vi "ZM_valve_state.vi"(0 "Z_Source":T1(ring), 1 "Z_State":T2(ring), 2 "open":bool, 3 "close":bool, 7 "T_start_delay":u32=300, 9 "T_stop_delay":u32=300, 11 "T_restart_delay":u32=3000) -> (14 "Start":bool, 15 "Stop":bool, 16 "End":bool, 17 "ZM_State":u32, 18 "t":u32)   [LabVIEW 2019, in "Valves.lvlib"]
uses:
  Valves.lvlib
  Trigers/RS.vi
  Timer Delay/Timer.vi
  Userlib.lvlib
panel:
  in  "t2_tmp":u32[][](array[numeric])=[[0, 0], [0, 0], [0, 0], [0, 0], [0, 0], [0, 0], [0, 0], [0, 0], [0, 0], [0, 0], [0, 0], [0, 0], [0, 0]]
  in  "C2_tmp":cluster{"C":bool, "NC":u32}[][](array[cluster])
  in  "t_tmp":u32[][](array[numeric])=[[0, 0], [0, 0], [0, 0], [0, 0], [0, 0], [0, 0], [0, 0], [0, 0], [0, 0], [0, 0], [0, 0], [0, 0], [0, 0]]
  in  "C_tmp":cluster{"C":bool, "NC":u32}[][](array[cluster])
  # "Temporally arrays"
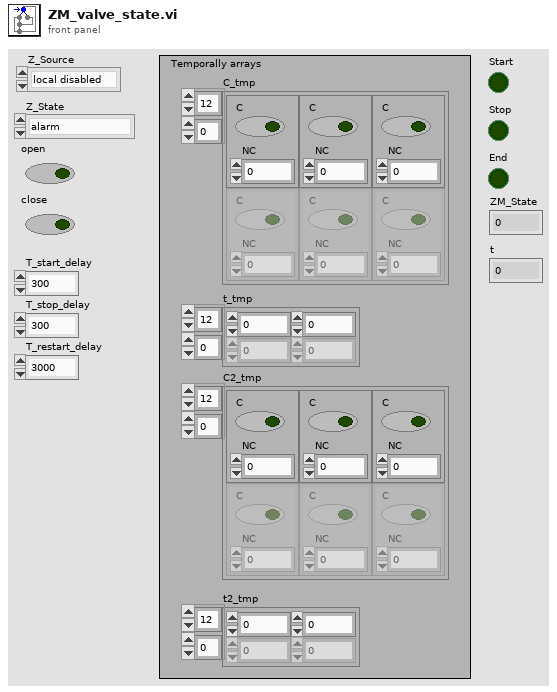
[diagram p1: front panel]
types:
  T1 = enum8{"local disabled", "local hand", "hand", "auto", "dist"}
  T2 = enum8{"alarm", "disabled", "not ready", "stop ready", "reserv", "switched off", "switched on", "check", "on min", "decrease speed", "on", "increase speed", "on max"}
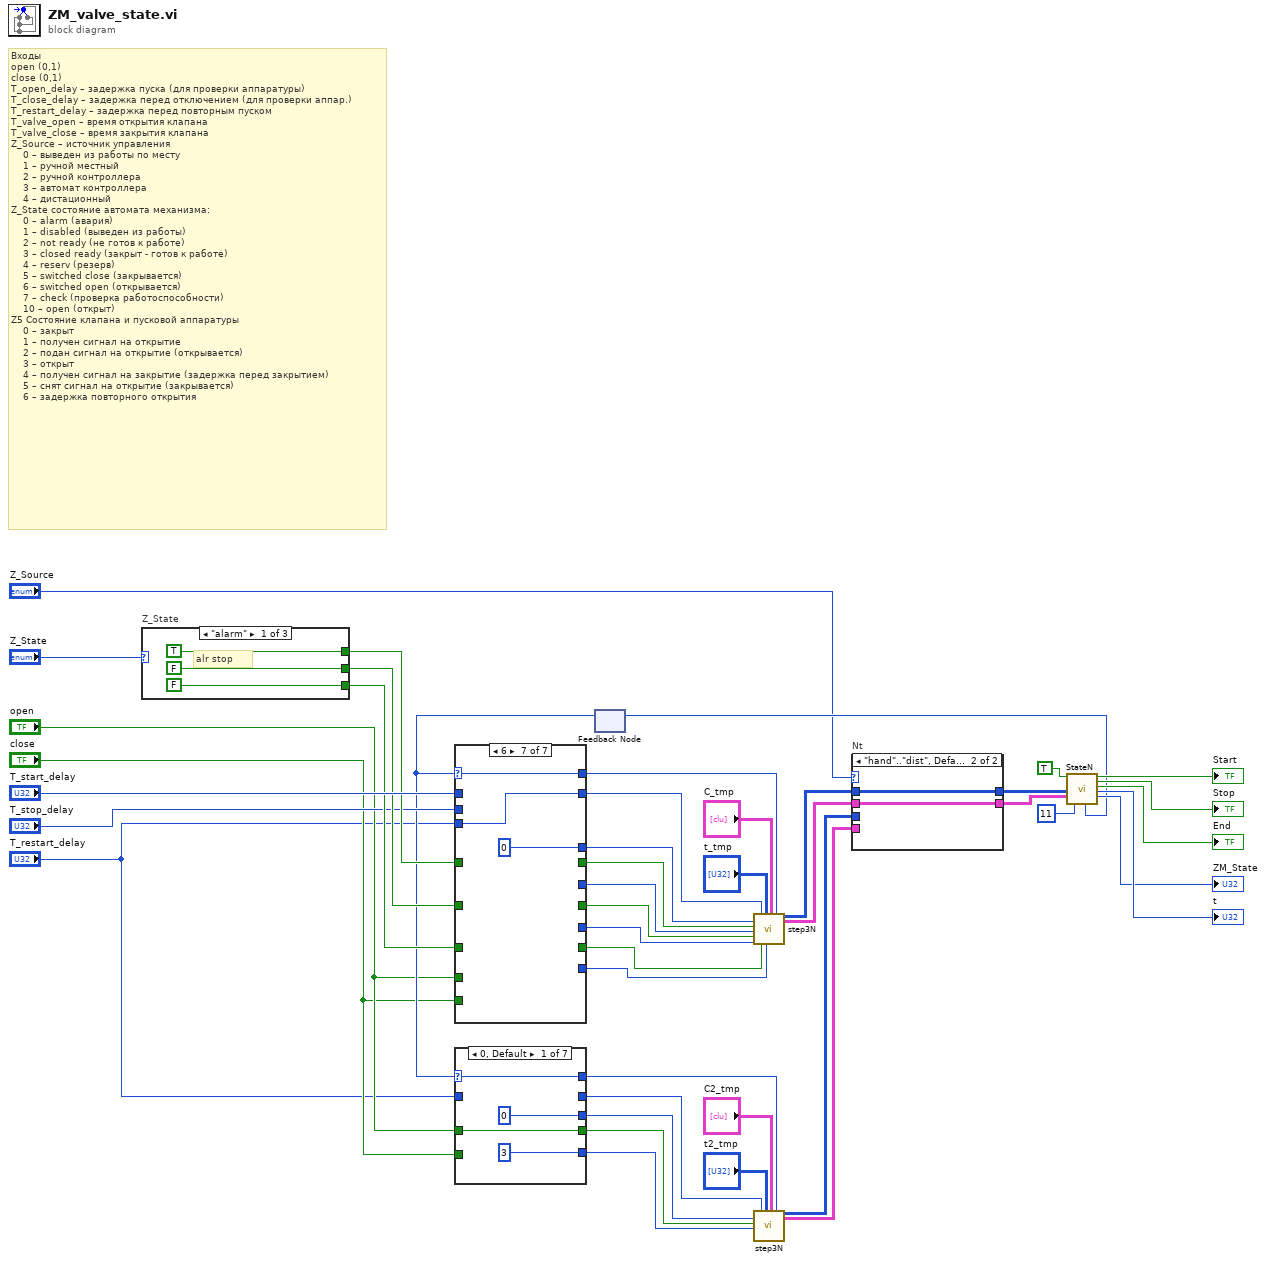
[diagram p0: block diagram]
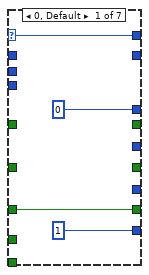
[diagram p2: hidden frame]
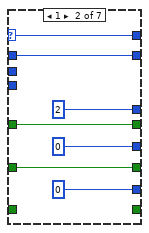
[diagram p3: hidden frame]
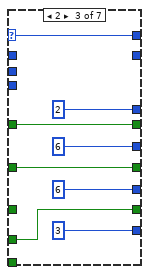
[diagram p4: hidden frame]
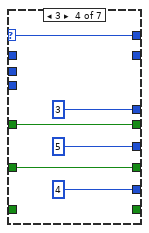
[diagram p5: hidden frame]
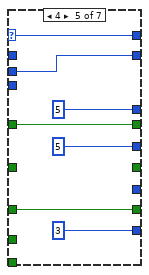
[diagram p6: hidden frame]
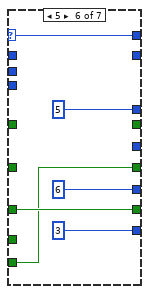
[diagram p7: hidden frame]
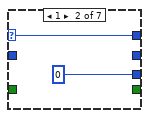
[diagram p8: hidden frame]
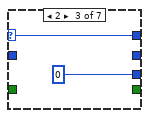
[diagram p9: hidden frame]
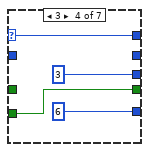
[diagram p10: hidden frame]
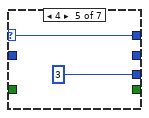
[diagram p11: hidden frame]
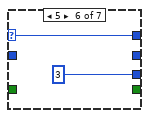
[diagram p12: hidden frame]
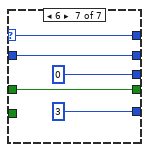
[diagram p13: hidden frame]
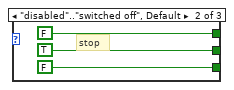
[diagram p15: hidden frame]
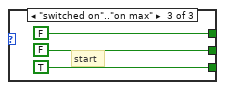
[diagram p16: hidden frame]
diagram:
  # "Входы\nopen (0,1)\nclose (0,1)\nT_open_delay – задержка пуска (для проверки аппаратуры)\nT_close_delay – задержка перед отключением (для проверки аппар.)\nT_restart_delay – задержка перед повторным пуском\nT_valve_open – время открытия клапана\nT_valve_close – время закрытия клапана\nZ_Source – источник управления\n    0 – выведен из работы по месту\n    1 – ручной местный\n    2 – ручной контроллера\n    3 – автомат контроллера\n    4 – дистационный\nZ_State состояние автомата механизма:\n    0 – alarm (авария)\n    1 – disabled (выведен из работы)\n    2 – not ready (не готов к работе)\n    3 – closed ready (закрыт - готов к работе)\n    4 – reserv (резерв)\n    5 – switched close (закрывается)\n    6 – switched open (открывается)\n    7 – check (проверка работоспособности)\n    10 – open (открыт)\nZ5 Состояние клапана и пусковой аппаратуры\n    0 – закрыт\n    1 – получен сигнал на открытие\n    2 – подан сигнал на открытие (открывается)\n    3 – открыт\n    4 – получен сигнал на закрытие (задержка перед закрытием)\n    5 – снят сигнал на открытие (закрывается)\n    6 – задержка повторного открытия"
  n1 = case "Z_State" shown="\"alarm\"" "Z_State" {
    tunnel: [FALSE TRUE FALSE] -> w25
    tunnel: [FALSE FALSE TRUE] -> w27
    tunnel: [TRUE FALSE FALSE] -> w24
    frame "alarm" {
      # "alr stop"
    }
    frame "disabled".."switched off", Default {
      # "stop"
    }
    frame "switched on".."on max" {
      # "start"
    }
  }
  n2 = feedback #1() -> (w11:u32)  [unwired: 1 in]
  n3 = case shown="6" w11 {
    selector: w11 -> [w56 w63 w71 w77 w84 w90 w93]
    tunnel: "T_start_delay" -> [_ w57 _ _ _ _ _]
    tunnel: [w56 w63 w71 w77 w84 w90 w93] -> w20
    tunnel: [u32 0 ("End step") u32 2 ("End step") u32 2 ("End step") u32 3 ("End step") u32 5 ("End step") u32 5 ("End step") u32 0 ("End step")] -> w32
    tunnel: [_ w57 _ _ w78 _ w91] -> w31
    tunnel: [_ w59 w66 w73 w81 _ _] -> w30
    tunnel: [_ u32 0 ("End step") u32 6 ("End step") u32 5 ("End step") u32 5 ("End step") _ _] -> w29
    tunnel: [w54 _ w64 _ w79 w86 _] -> w28
    tunnel: w27 -> [w54 _ _ _ w79 w86 _]
    tunnel: [u32 1 ("End step") _ u32 3 ("End step") _ u32 3 ("End step") u32 3 ("End step") _] -> w26
    tunnel: w25 -> [_ w61 w68 w75 _ _ _]
    tunnel: [_ w61 w68 w75 _ w85 _] -> w23
    tunnel: [_ u32 0 ("End step") u32 6 ("End step") u32 4 ("End step") _ u32 6 ("End step") _] -> w22
    tunnel: w24 -> [_ w59 w66 w73 w81 _ _]
    tunnel: "open" -> [_ _ w64 _ _ _ _]
    tunnel: "T_stop_delay" -> [_ _ _ _ w78 _ _]
    tunnel: "close" -> [_ _ _ _ _ w85 _]
    tunnel: "T_restart_delay" -> [_ _ _ _ _ _ w91]
    frame 0, Default {
    }
    frame 1 {
    }
    frame 2 {
    }
    frame 3 {
    }
    frame 4 {
    }
    frame 5 {
    }
    frame 6 {
    }
  }
  n4 = case shown="0, Default" w11 {
    selector: w11 -> [w97 w99 w101 w105 w107 w109 w114]
    tunnel: [w97 w99 w101 w105 w107 w109 w114] -> w16
    tunnel: [u32 0 ("End step") u32 0 ("End step") u32 0 ("End step") u32 3 ("End step") u32 3 ("End step") u32 3 ("End step") u32 0 ("End step")] -> w12
    tunnel: [_ _ _ _ _ _ w112] -> w13
    tunnel: [w95 _ _ w102 _ _ w111] -> w14
    tunnel: [u32 3 ("End step") _ _ u32 6 ("End step") _ _ u32 3 ("End step")] -> w15
    tunnel: "open" -> [w95 _ _ _ _ _ w111]
    tunnel: "close" -> [_ _ _ w102 _ _ _]
    tunnel: "T_restart_delay" -> [_ _ _ _ _ _ w112]
    frame 0, Default {
    }
    frame 1 {
    }
    frame 2 {
    }
    frame 3 {
    }
    frame 4 {
    }
    frame 5 {
    }
    frame 6 {
    }
  }
  n5 = call "step3N.vi"("NT"=w32, "C1"=w30, "NC1"=w29, "C2"=w23, "NC2"=w22, "T"=w31, "C3"=w28, "T NT2"="t_tmp", "NC3"=w26, "C NC2"="C_tmp", "N step"=w20) -> ("T NT"=w18:u32[][], "C NC"=w17:cluster{"C":bool, "NC":u32}[][])  [unwired: 7 in]
  n6 = call "step3N.vi"("NT"=w12, "C1"=w14, "NC1"=w15, "T"=w13, "T NT2"="t2_tmp", "C NC2"="C2_tmp", "N step"=w16) -> ("T NT"=w6:u32[][], "C NC"=w5:cluster{"C":bool, "NC":u32}[][])  [unwired: 11 in]
  n7 = case "Nt" shown="\"hand\"..\"dist\", Default" "Z_Source" {
    tunnel: w18 -> [_ w118]
    tunnel: w17 -> [_ w117]
    tunnel: [w116 w118] -> w37
    tunnel: [w115 w117] -> w36
    tunnel: w6 -> [w116 _]
    tunnel: w5 -> [w115 _]
    frame "local disabled", "local hand" {
    }
    frame "hand".."dist", Default {
    }
  }
  n8 = call "StateN.vi"("Start"=TRUE, "T_table"=w37, "C_table"=w36, "End step"=u32 11) -> ("N next"=w19:u32, "Start"=→"Start":bool, "Stop"=→"Stop":bool, "End"=→"End":bool, "t"=→"t":u32, "N curr"=→"ZM_State":u32)  [unwired: 10 in]
  n9 = feedback-in #1(w19) -> ()
